vi "advance_waveform_part.vi"(8 "Ramp parameters":T2, 9 "Cycle parameters":T6, 10 "Cycle counters in":T7, 11 "Scan counters in":T8 {"Current part of waveform" items=["Imaging", "Settling", "Resting"]}) -> (1 "Current ramp values":T1, 2 "Cycle counters out":T7, 3 "Scan counters out":T8 {"Current part of waveform" items=["Imaging", "Settling", "Resting"]})   [LabVIEW 2011]
uses:
  typedefs/scan_counters_cluster.ctl
  typedefs/cycle_counters_cluster.ctl
  typedefs/cycle_parameters_cluster.ctl
  typedefs/ramp_parameters_cluster.ctl
  typedefs/ramp_type_enum.ctl
  typedefs/linear_ramp_parameters_cluster.ctl
  typedefs/sine_ramp_parameters_cluster.ctl
  typedefs/current_ramp_values_cluster.ctl
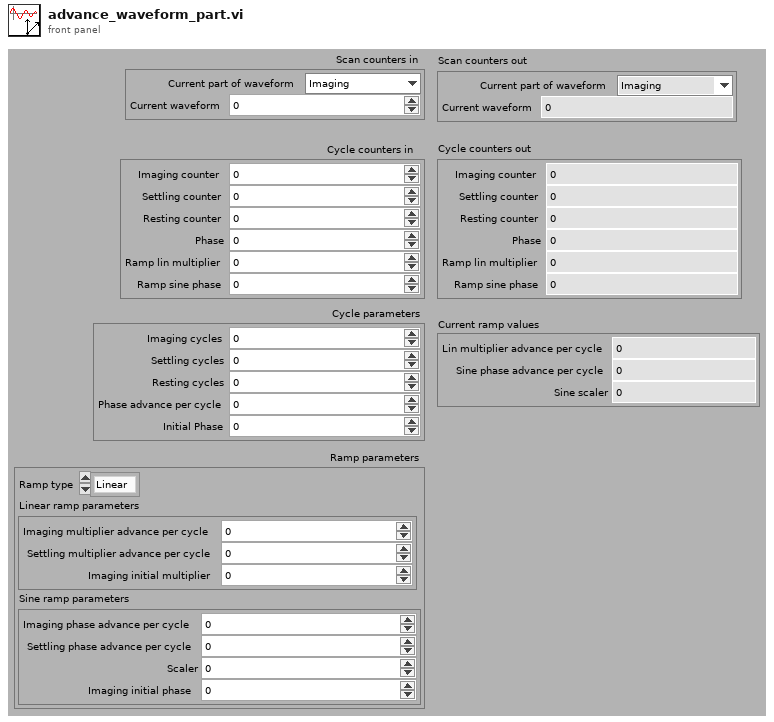
[diagram p1: front panel]
types:
  T1 = typedef "current_ramp_values_cluster.ctl" = cluster{"Lin multiplier advance per cycle":fxp<+/-,32,0>, "Sine phase advance per cycle":fxp<+,32,0>, "Sine scaler":fxp<+,43,12>}
  T2 = typedef "ramp_parameters_cluster.ctl" = cluster{"Ramp type":T3, "Linear ramp parameters":T4, "Sine ramp parameters":T5}
  T3 = typedef "ramp_type_enum.ctl" = enum8{"Linear", "Sine"}
  T4 = typedef "linear_ramp_parameters_cluster.ctl" = cluster{"Imaging multiplier advance per cycle":fxp<+/-,32,0>, "Settling multiplier advance per cycle":fxp<+/-,32,0>, "Imaging initial multiplier":fxp<+/-,43,12>}
  T5 = typedef "sine_ramp_parameters_cluster.ctl" = cluster{"Imaging phase advance per cycle":fxp<+,32,0>, "Settling phase advance per cycle":fxp<+,32,0>, "Scaler":fxp<+,43,12>, "Imaging initial phase":fxp<+,32,1>}
  T6 = typedef "cycle_parameters_cluster.ctl" = cluster{"Imaging cycles":i32, "Settling cycles":i32, "Resting cycles":i32, "Phase advance per cycle":fxp<+,32,0>, "Initial Phase":fxp<+,32,1>}
  T7 = typedef "cycle_counters_cluster.ctl" = cluster{"Imaging counter":i32, "Settling counter":i32, "Resting counter":i32, "Phase":fxp<+,32,1>, "Ramp lin multiplier":fxp<+/-,43,12>, "Ramp sine phase":fxp<+,32,1>}
  T8 = typedef "scan_counters_cluster.ctl" = cluster{"Current part of waveform":u8, "Current waveform":u16}
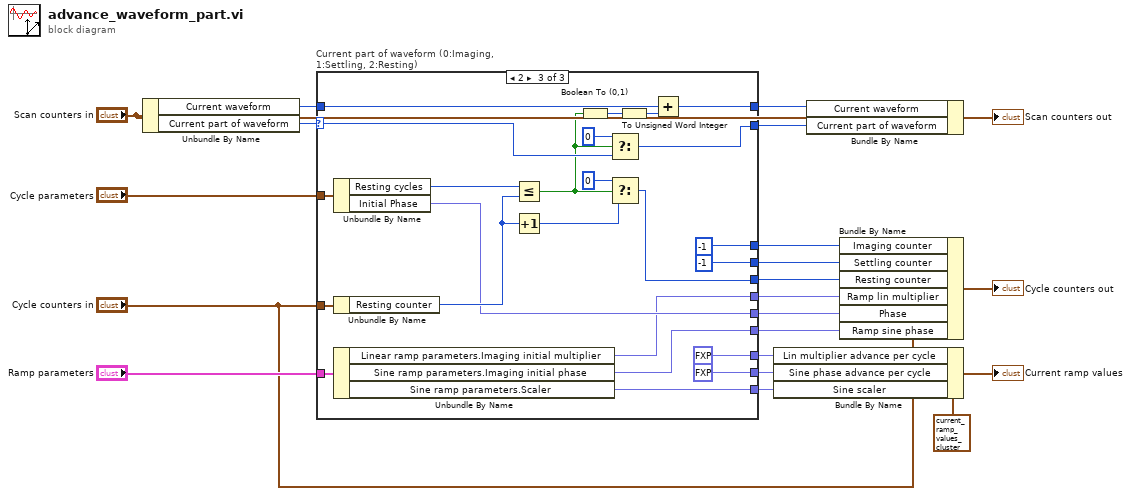
[diagram p0: block diagram]
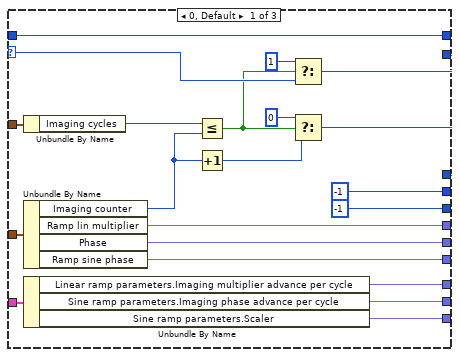
[diagram p2: hidden frame]
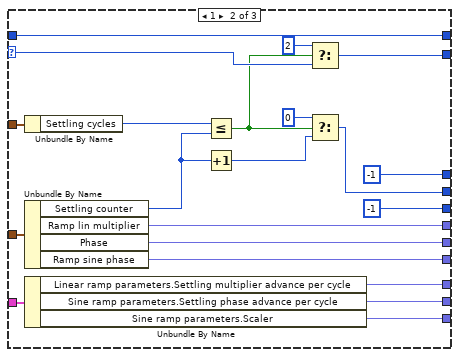
[diagram p3: hidden frame]
diagram:
  n1 = Unbundle By Name("Scan counters in") -> ("Current waveform"=w21:u16, "Current part of waveform"=w20:u8)
  n2 = case "Current part of waveform (0:Imaging, 1:Settling, 2:Resting)" shown="2" w20 {
    selector: w20 -> [w42 w62 w86]
    tunnel: [w40 w61 w85] -> w18
    tunnel: w21 -> [w39 w60 w84]
    tunnel: [w39 w60 w83] -> w19
    tunnel: "Cycle parameters" -> [w31 w52 w80]
    tunnel: "Cycle counters in" -> [w38 w54 w79]
    tunnel: [w37 w56 w66] -> w16
    tunnel: [w33 w55 w75] -> w15
    tunnel: [w25 w46 fxp<+/-,32,0> 0.0 ("Settling Multiplier advance per cycle")] -> w5
    tunnel: [w27 -1 ("Imaging counter") -1 ("Imaging counter")] -> w11
    tunnel: [-1 ("t") w48 -1 ("t")] -> w10
    tunnel: [-1 ("t") -1 ("t") w71] -> w9
    tunnel: "Ramp parameters" -> [w26 w47 w67]
    tunnel: [w24 w45 fxp<+,32,0> 0.0 ("Settling phase advance per cycle")] -> w4
    tunnel: [w23 w44 w64] -> w3
    tunnel: [w22 w43 w65] -> w6
    frame 0, Default {
      n3 = Unbundle By Name(w31) -> ("Imaging cycles"=w36:i32)
      n4 = Unbundle By Name(w38) -> ("Imaging counter"=w30:i32, "Ramp lin multiplier"=w37:fxp<+/-,43,12>, "Phase"=w33:fxp<+,32,1>, "Ramp sine phase"=w22:fxp<+,32,1>)
      n5 = Unbundle By Name(w26) -> ("Linear ramp parameters.Imaging multiplier advance per cycle"=w25:fxp<+/-,32,0>, "Sine ramp parameters.Imaging phase advance per cycle"=w24:fxp<+,32,0>, "Sine ramp parameters.Scaler"=w23:fxp<+,43,12>)
      n6 = Less Or Equal?(x=w36, y=w30) -> (x <= y?=w32:bool)
      n7 = Increment(x=w30) -> (x+1=w35:i32)
      n8 = Select(t=u8 1, s=w32, f=w42) -> (s? t:f=w40:u8)
      n9 = Select(t=0, s=w32, f=w35) -> (s? t:f=w27:i32)
    }
    frame 1 {
      n10 = Unbundle By Name(w52) -> ("Settling cycles"=w59:i32)
      n11 = Unbundle By Name(w54) -> ("Settling counter"=w51:i32, "Ramp lin multiplier"=w56:fxp<+/-,43,12>, "Phase"=w55:fxp<+,32,1>, "Ramp sine phase"=w43:fxp<+,32,1>)
      n12 = Unbundle By Name(w47) -> ("Linear ramp parameters.Settling multiplier advance per cycle"=w46:fxp<+/-,32,0>, "Sine ramp parameters.Settling phase advance per cycle"=w45:fxp<+,32,0>, "Sine ramp parameters.Scaler"=w44:fxp<+,43,12>)
      n13 = Less Or Equal?(x=w59, y=w51) -> (x <= y?=w53:bool)
      n14 = Increment(x=w51) -> (x+1=w58:i32)
      n15 = Select(t=u8 2, s=w53, f=w62) -> (s? t:f=w61:u8)
      n16 = Select(t=0, s=w53, f=w58) -> (s? t:f=w48:i32)
    }
    frame 2 {
      n17 = Unbundle By Name(w80) -> ("Resting cycles"=w82:i32, "Initial Phase"=w75:fxp<+,32,1>)
      n18 = Unbundle By Name(w79) -> ("Resting counter"=w78:i32)
      n19 = Unbundle By Name(w67) -> ("Linear ramp parameters.Imaging initial multiplier"=w66:fxp<+/-,43,12>, "Sine ramp parameters.Imaging initial phase"=w65:fxp<+,32,1>, "Sine ramp parameters.Scaler"=w64:fxp<+,43,12>)
      n20 = Less Or Equal?(x=w82, y=w78) -> (x <= y?=w77:bool)
      n21 = Increment(x=w78) -> (x+1=w72:i32)
      n22 = Boolean To (0,1)(Boolean=w77) -> (0, 1=w69:i16)
      n23 = Select(t=u8 0, s=w77, f=w86) -> (s? t:f=w85:u8)
      n24 = Select(t=0, s=w77, f=w72) -> (s? t:f=w71:i32)
      n25 = To Unsigned Word Integer(number=w69) -> (unsigned 16bit integer=w70:u16)
      n26 = Add(x=w84, y=w70) -> (x+y=w83:u16)
    }
  }
  n27 = Bundle By Name(cluster=T1 {"Lin multiplier advance per cycle"=0.0, "Sine phase advance per cycle"=0.0, "Sine scaler"=0.0} ("Current ramp values 2"), "Lin multiplier advance per cycle"=w5, "Sine phase advance per cycle"=w4, "Sine scaler"=w3) -> (→"Current ramp values":T1)
  n28 = Bundle By Name(cluster="Scan counters in", "Current waveform"=w19, "Current part of waveform"=w18) -> (→"Scan counters out":T8)
  n29 = Bundle By Name(cluster="Cycle counters in", "Imaging counter"=w11, "Settling counter"=w10, "Resting counter"=w9, "Ramp lin multiplier"=w16, "Phase"=w15, "Ramp sine phase"=w6) -> (→"Cycle counters out":T7)
